vi "IMAQ FPGA Camera Link Pixel Packer U8x10.vi"(8 "Input Valid":bool, 9 "Frame Valid In":bool, 10 "Line Valid In":bool, 11 "Pixels In":u8[](array[numeric])=[0, 0, 0, 0, 0, 0, 0, 0, 0, 0]) -> (0 "Output Valid":bool, 1 "Frame Valid Out":bool, 2 "Line Valid Out":bool, 3 "Pixel Bus x8 Out":cluster{"Pixels":u8[], "DV":bool[]}, 5 "Overflow":bool)   [LabVIEW 2020]
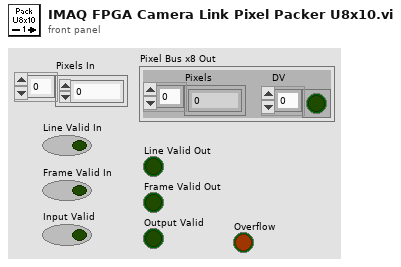
[diagram p1: front panel]
types:
  T1 = enum16{"Wait to Pack", "Pack", "Pack Last Items", "Add EOL", "Add EOI"}
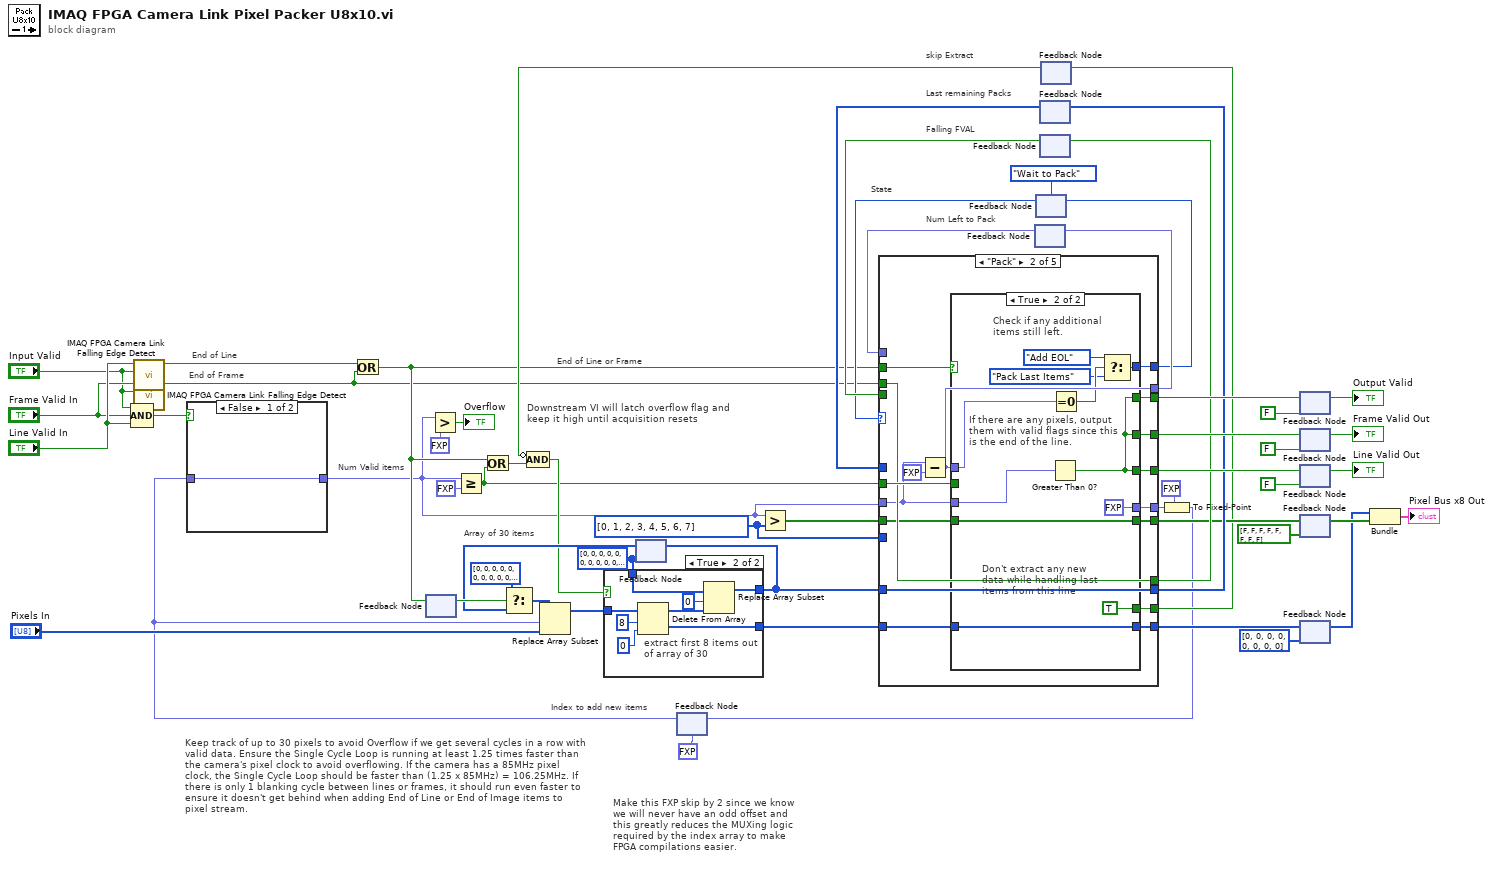
[diagram p0: block diagram]
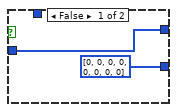
[diagram p2: hidden frame]
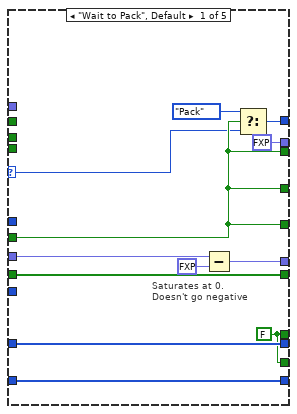
[diagram p3: hidden frame]
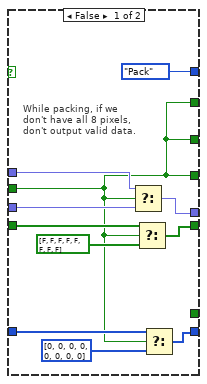
[diagram p4: hidden frame]
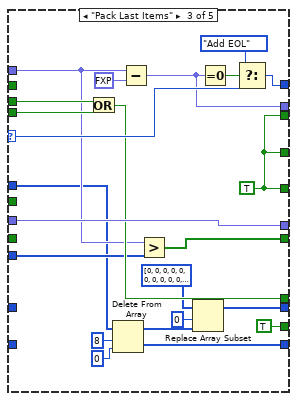
[diagram p5: hidden frame]
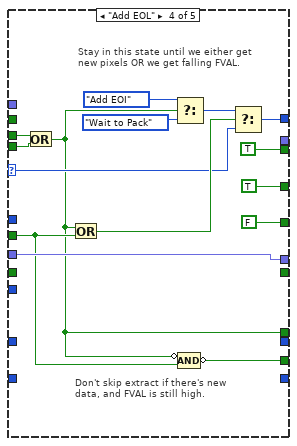
[diagram p6: hidden frame]
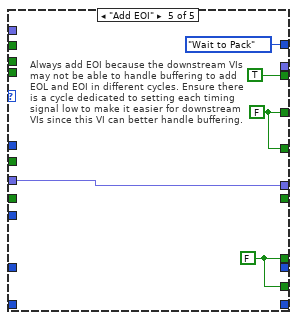
[diagram p7: hidden frame]
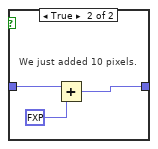
[diagram p8: hidden frame]
diagram:
  w22 = i16[] [0, 1, 2, 3, 4, 5, 6, 7]
  w29 = u8[] [0, 0, 0, 0, 0, 0, 0, 0, 0, 0, 0, 0, 0, 0, 0, 0, 0, 0, 0, 0, 0, 0, 0, 0, 0, 0, 0, 0, 0, 0] ("Array of 30 Pixels")
  # "End of Line"
  # "skip Extract"
  # "Last remaining Packs"
  # "End of Frame"
  # "End of Line or Frame"
  # "Make this FXP skip by 2 since we know we will never have an odd offset and this greatly reduces the MUXing logic required by the index array to make FPGA compilations easier."
  # "Array of 30 items"
  # "Falling FVAL"
  # "Num Left to Pack"
  # "State"
  # "Downstream VI will latch overflow flag and keep it high until acquisition resets"
  # "Keep track of up to 30 pixels to avoid Overflow if we get several cycles in a row with valid data. Ensure the Single Cycle Loop is running at least 1.25 times faster than the camera's pixel clock to avoid overflowing. If the camera has a 85MHz pixel clock, the Single Cycle Loop should be faster than (1.25 x 85MHz) = 106.25MHz. If there is only 1 blanking cycle between lines or frames, it should run even faster to ensure it doesn't get behind when adding End of Line or End of Image items to pixel stream."
  # "Num Valid items"
  # "Index to add new items"
  n1 = Compound Arithmetic op=AND("Input Valid", "Frame Valid In", "Line Valid In") -> (w45:bool)
  n2 = call <vilib>:"IMAQ FPGA Camera Link Falling Edge Detect.vi"("Input Valid"="Input Valid", "Input"="Line Valid In") -> ("Falling Edge"=w36:bool)  [unwired: 9 in]
  n3 = call <vilib>:"IMAQ FPGA Camera Link Falling Edge Detect.vi"("Input Valid"="Input Valid", "Input"="Frame Valid In") -> ("Falling Edge"=w6:bool)  [unwired: 9 in]
  n4 = Or(x=w36, y=w6) -> (x .or. y?=w7:bool)
  n5 = feedback #1() -> (w19:bool)  [unwired: 1 in]
  n6 = feedback-in #1(w7) -> ()
  n7 = feedback #2(w29) -> (w18:u8[])
  n8 = Select(t=u8[] [0, 0, 0, 0, 0, 0, 0, 0, 0, 0, 0, 0, 0, 0, 0, 0, 0, 0, 0, 0, 0, 0, 0, 0, 0, 0, 0, 0, 0, 0] ("Array of 30 Pixels"), s=w19, f=w18) -> (s? t:f=w17:u8[])
  n9 = feedback #3(fxp<+,4,5> 0.0) -> (w37:fxp<+,4,5>)
  n10 = case shown="False" w45 {
    tunnel: w37 -> [w58 w61]
    tunnel: [w58 w60] -> w4
    frame False {
    }
    frame True {
      # "We just added 10 pixels."
      n11 = Add(x=w61, y=fxp<+,4,5> 10.0) -> (x+y=w60:fxp<+,5,6>)
    }
  }
  n12 = Greater?(x=w4, y=fxp<+,4,5> 30.0) -> (0:→"Overflow":bool)
  n13 = Greater Or Equal?(x=w4, y=fxp<+,4,5> 8.0) -> (x >= y?=w5:bool)
  n14 = Or(x=w7, y=w5) -> (x .or. y?=w20:bool)
  n15 = Replace Array Subset(array=w17, new element="Pixels In", index=w37) -> (w41:u8[])
  n16 = Greater?(x=w4, y=w22) -> (0:w3:bool[])
  n17 = feedback #4() -> (w9:fxp<+,5,6>)  [unwired: 1 in]
  n18 = feedback #5(T1."Wait to Pack") -> (w10:T1)
  n19 = feedback #6() -> (w8:u8[])  [unwired: 1 in]
  n20 = feedback #7() -> (w26:bool)  [unwired: 1 in]
  n21 = feedback #8() -> (w21:bool)  [unwired: 1 in]
  n22 = Compound Arithmetic op=AND(invert w21, w20) -> (w15:bool)
  n23 = case shown="True" w15 {
    tunnel: w41 -> [w63 w71]
    tunnel: w29 -> [_ w68]
    tunnel: [u8[] [0, 0, 0, 0, 0, 0, 0, 0] ("Array of 30 Pixels") w67] -> w1
    tunnel: [w63 w66] -> w2
    frame False {
    }
    frame True {
      # "extract first 8 items out of array of 30"
      n24 = Delete From Array(array=w71, length=8, index=0) -> (deleted portion=w67:u8[], array with subset deleted=w70:u8[])
      n25 = Replace Array Subset(array=w68, new element=w70, index=0) -> (w66:u8[])
    }
  }
  n26 = feedback-in #2(w2) -> ()
  n27 = case shown="\"Pack\"" w10 {
    selector: w10 -> [w80 _ w145 w150 _]
    tunnel: w4 -> [w78 w92 w140 w156 w162]
    tunnel: [w77 w95 w140 w156 w162] -> w12
    tunnel: [w83 w99 w142 FALSE w163] -> w34
    tunnel: [w83 w98 w142 TRUE w163] -> w33
    tunnel: [w83 w97 w142 TRUE TRUE] -> w32
    tunnel: [w81 w96 w144 w157 T1."Wait to Pack"] -> w30
    tunnel: w7 -> [_ w91 _ _ _]
    tunnel: [fxp<+,4,5> 0.0 w89 w123 _ _] -> w31
    tunnel: w9 -> [_ _ w135 _ _]
    tunnel: w2 -> [w76 w86 _ _ _]
    tunnel: w5 -> [w83 w100 _ w148 _]
    tunnel: [w76 w86 w124 _ _] -> w28
    tunnel: w8 -> [_ _ w129 _ _]
    tunnel: w6 -> [_ w94 w138 w159 _]
    tunnel: [w72 w94 w137 w147 w161] -> w27
    tunnel: w26 -> [_ _ w139 w158 _]
    tunnel: w1 -> [w75 w85 _ _ _]
    tunnel: [w75 w84 w128 _ _] -> w25
    tunnel: w3 -> [w74 w88 _ _ _]
    tunnel: [w74 w87 w133 _ _] -> w24
    tunnel: [w72 w90 TRUE ("Falling Edge") w146 w161] -> w23
    tunnel: w22 -> [_ _ w134 _ _]
    frame "Wait to Pack", Default {
      w72 = FALSE ("Falling Edge")
      # "Saturates at 0. Doesn't go negative"
      n28 = Subtract(x=w78, y=fxp<+,4,5> 8.0) -> (x-y=w77:fxp<+,5,6>)
      n29 = Select(t=T1."Pack", s=w83, f=w80) -> (s? t:f=w81:T1)
    }
    frame "Pack" {
      n30 = Subtract(x=w92, y=fxp<+,4,5> 8.0) -> (x-y=w89:fxp<+,5,6>)
      n31 = case shown="True" w91 {
        tunnel: w100 -> [w102 _]
        tunnel: [w102 w117] -> w99
        tunnel: [w102 w117] -> w98
        tunnel: [w102 w117] -> w97
        tunnel: [T1."Pack" w119] -> w96
        tunnel: w92 -> [w110 w118]
        tunnel: [w109 fxp<+,5,6> 0.0] -> w95
        tunnel: w89 -> [w108 w115]
        tunnel: [_ TRUE] -> w90
        tunnel: w88 -> [w107 w114]
        tunnel: [w106 w114] -> w87
        tunnel: w85 -> [w104 w113]
        tunnel: [w103 w113] -> w84
        frame False {
          # "While packing, if we don't have all 8 pixels, don't output valid data."
          n32 = Select(t=w108, s=w102, f=w110) -> (s? t:f=w109:fxp<+,5,6>)
          n33 = Select(t=w107, s=w102, f=bool[] [FALSE, FALSE, FALSE, FALSE, FALSE, FALSE, FALSE, FALSE]) -> (s? t:f=w106:bool[])
          n34 = Select(t=w104, s=w102, f=u8[] [0, 0, 0, 0, 0, 0, 0, 0]) -> (s? t:f=w103:u8[])
        }
        frame True {
          # "Check if any additional items still left."
          # "If there are any pixels, output them with valid flags since this is the end of the line."
          # "Don't extract any new data while handling last items from this line"
          n35 = Greater Than 0?(x=w118) -> (x > 0?=w117:bool)
          n36 = Equal To 0?(x=w115) -> (x = 0?=w122:bool)
          n37 = Select(t=T1."Add EOL", s=w122, f=T1."Pack Last Items") -> (s? t:f=w119:T1)
        }
      }
    }
    frame "Pack Last Items" {
      w142 = TRUE
      n38 = Or(x=w138, y=w139) -> (x .or. y?=w137:bool)
      n39 = Delete From Array(array=w129, length=8, index=0) -> (deleted portion=w128:u8[], array with subset deleted=w125:u8[])
      n40 = Subtract(x=w135, y=fxp<+,4,5> 8.0) -> (x-y=w123:fxp<+,5,6>)
      n41 = Greater?(x=w135, y=w134) -> (0:w133:bool[])
      n42 = Replace Array Subset(array=u8[] [0, 0, 0, 0, 0, 0, 0, 0, 0, 0, 0, 0, 0, 0, 0, 0, 0, 0, 0, 0, 0, 0, 0, 0, 0, 0, 0, 0, 0, 0] ("Array of 30 Pixels"), new element=w125, index=0) -> (w124:u8[])
      n43 = Equal To 0?(x=w123) -> (x = 0?=w141:bool)
      n44 = Select(t=T1."Add EOL", s=w141, f=w145) -> (s? t:f=w144:T1)
    }
    frame "Add EOL" {
      # "Don't skip extract if there's new data, and FVAL is still high."
      # "Stay in this state until we either get new pixels OR we get falling FVAL."
      n45 = Or(x=w159, y=w158) -> (x .or. y?=w147:bool)
      n46 = Or(x=w147, y=w148) -> (x .or. y?=w152:bool)
      n47 = Select(t=T1."Add EOI", s=w147, f=T1."Wait to Pack") -> (s? t:f=w151:T1)
      n48 = Compound Arithmetic op=AND(invert w147, w148) -> (invert w146:bool)
      n49 = Select(t=w151, s=w152, f=w150) -> (s? t:f=w157:T1)
    }
    frame "Add EOI" {
      w161 = FALSE ("Falling Edge")
      w163 = FALSE
      # "Always add EOI because the downstream VIs may not be able to handle buffering to add EOL and EOI in different cycles. Ensure there is a cycle dedicated to setting each timing signal low to make it easier for downstream VIs since this VI can better handle buffering."
    }
  }
  n50 = feedback-in #4(w31) -> ()
  n51 = feedback-in #5(w30) -> ()
  n52 = feedback-in #6(w28) -> ()
  n53 = feedback-in #7(w27) -> ()
  n54 = feedback-in #8(w23) -> ()
  n55 = To Fixed-Point(fixed-point type=fxp<+,4,5> 0.0, number=w12) -> (fixed-point=w11:fxp<+,4,5>)
  n56 = feedback-in #3(w11) -> ()
  n57 = feedback #9(FALSE) -> (→"Output Valid":bool)
  n58 = feedback-in #9(w32) -> ()
  n59 = feedback #10(FALSE) -> (→"Frame Valid Out":bool)
  n60 = feedback-in #10(w33) -> ()
  n61 = feedback #11(FALSE) -> (→"Line Valid Out":bool)
  n62 = feedback-in #11(w34) -> ()
  n63 = feedback #12(bool[] [FALSE, FALSE, FALSE, FALSE, FALSE, FALSE, FALSE, FALSE]) -> (w50:bool[])
  n64 = feedback-in #12(w24) -> ()
  n65 = feedback #13(u8[] [0, 0, 0, 0, 0, 0, 0, 0] ("Pixels")) -> (w49:u8[])
  n66 = feedback-in #13(w25) -> ()
  n67 = Bundle("Pixels"=w49, w50) -> (→"Pixel Bus x8 Out":cluster{"Pixels":u8[], bool[]})  [unwired: 1 in]
